vi "calc polar angles for unit vector start.vi"(10 "unit vector in":T1={"nx"=0.54, "ny"=0.6, "nz"=0.6}) -> (0 "signal valid":bool=TRUE, 1 "checksum":sgl=1.0057833, 2 "polar angles out":T2={"theta [degrees]"=53.37679, "phi [degrees]"=48.012787})   [LabVIEW 2014]
doc: "Calc Polar Angles for Unit Vector\n\nInputs a unit vector and outputs angles in polar form, while also indicating if the sensor detected a valid source.\n\nCalculations:\n\nphi = arctan(position along y-axis / position along x-axis) \ntheta = arctan (sqrt( (position along x-axis)^2 + (position along y -axis)^2) / (position along z-axis) )\nnxvalid (position along x is valid as sine or cosine) = True if -1 <= nx <= 1\nnyvalid (position along y is valid as sine or cosine) = True if -1 <= ny <= 1\nnzvalid (position along z is valid as sine or cosine) = True if -1 <= nz <= 1\n\n\n\nchecksum = sqrt( (position along x-axis)^2 + (position along y -axis)^2) / (position along z-axis)\nchecksumvalid (valid as unit 1 length) [bool] = True if 0.95 <= checksum <= 1.05, a 5% tolerance\nsignalvalid = nxvalid ^ nyvalid ^ nzvalid ^ checksumvalid\n\nBeverly Abadines\nPHY 350: E2"
uses:
  typedefs/polar angle typedef.ctl
  typedefs/unit vector typedef.ctl
panel:
  # "fully functional BD\n\nmake into a fully funtional subvi"
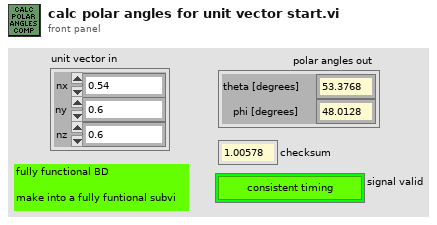
[diagram p1: front panel]
types:
  T1 = typedef "unit vector typedef.ctl" = cluster{"nx":sgl, "ny":sgl, "nz":sgl}
  T2 = typedef "polar angle typedef.ctl" = cluster{"theta [degrees]":sgl, "phi [degrees]":sgl}
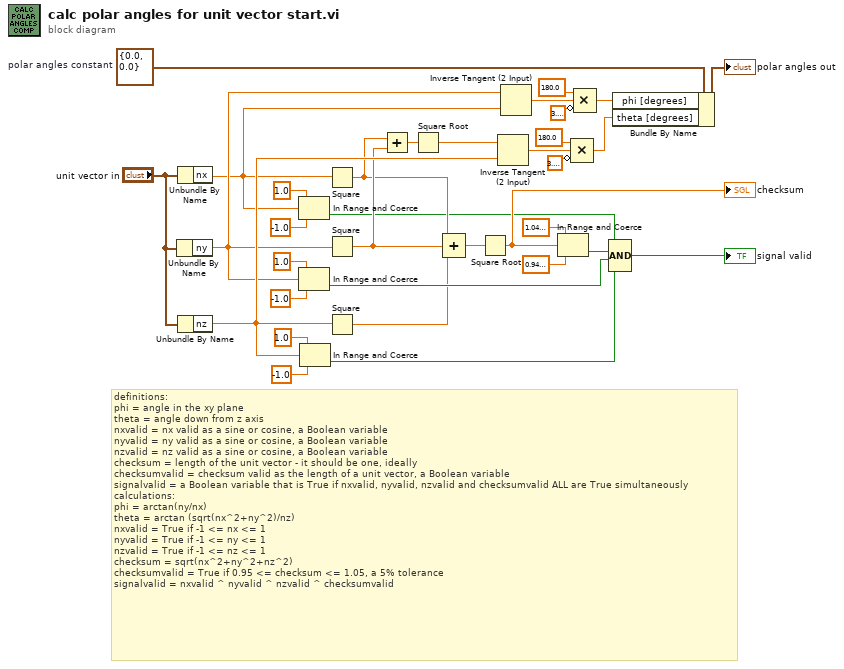
[diagram p0: block diagram]
diagram:
  w30 = T2 {"theta [degrees]"=0.0, "phi [degrees]"=0.0}  # polar angles constant
  # "definitions:\nphi = angle in the xy plane\ntheta = angle down from z axis\nnxvalid = nx valid as a sine or cosine, a Boolean variable \nnyvalid = ny valid as a sine or cosine, a Boolean variable\nnzvalid = nz valid as a sine or cosine, a Boolean variable\nchecksum = length of the unit vector - it should be one, ideally\nchecksumvalid = checksum valid as the length of a unit vector, a Boolean variable\nsignalvalid = a Boolean variable that is True if nxvalid, nyvalid, nzvalid and checksumvalid ALL are True simultaneously\ncalculations:\nphi = arctan(ny/nx)\ntheta = arctan (sqrt(nx^2+ny^2)/nz)\nnxvalid = True if -1 <= nx <= 1\nnyvalid = True if -1 <= ny <= 1\nnzvalid = True if -1 <= nz <= 1\nchecksum = sqrt(nx^2+ny^2+nz^2)\nchecksumvalid = True if 0.95 <= checksum <= 1.05, a 5% tolerance\nsignalvalid = nxvalid ^ nyvalid ^ nzvalid ^ checksumvalid"
  n1 = Unbundle By Name("unit vector in") -> ("ny"=w21:sgl)
  n2 = Unbundle By Name("unit vector in") -> ("nx"=w20:sgl)
  n3 = Unbundle By Name("unit vector in") -> ("nz"=w29:sgl)
  n4 = In Range and Coerce(upper limit=sgl 1.0, x=w20, lower limit=sgl -1.0) -> (In Range?=w15:bool)  [unwired: 1 out]
  n5 = In Range and Coerce(upper limit=sgl 1.0, x=w21, lower limit=sgl -1.0) -> (In Range?=w16:bool)  [unwired: 1 out]
  n6 = In Range and Coerce(upper limit=sgl 1.0, x=w29, lower limit=sgl -1.0) -> (In Range?=w17:bool)  [unwired: 1 out]
  n7 = Square(x=w20) -> (x^2=w22:sgl)
  n8 = Square(x=w21) -> (x^2=w23:sgl)
  n9 = Square(x=w29) -> (x^2=w11:sgl)
  n10 = Add(x=w22, y=w23) -> (x+y=w24:sgl)
  n11 = Square Root(x=w24) -> (sqrt(x)=w28:sgl)
  n12 = Compound Arithmetic op=ADD(w22, w23, w11) -> (w12:sgl)
  n13 = Square Root(x=w12) -> (sqrt(x)=w19:sgl)
  "checksum" <- w19
  n14 = Inverse Tangent (2 Input)(1:w29, 2:w28) -> (0:w27:sgl)
  n15 = Inverse Tangent (2 Input)(1:w20, 2:w21) -> (0:w1:sgl)
  n16 = In Range and Coerce(upper limit=sgl 1.05, x=w19, lower limit=sgl 0.95) -> (In Range?=w14:bool)  [unwired: 1 out]
  n17 = Compound Arithmetic op=MULTIPLY(sgl 180.0 ("value"), w27, invert sgl 3.1415927) -> (w33:sgl)
  n18 = Compound Arithmetic op=MULTIPLY(sgl 180.0 ("value"), w1, invert sgl 3.1415927) -> (w32:sgl)
  n19 = Compound Arithmetic op=AND(w15, w14, w16, w17) -> (→"signal valid":bool)
  n20 = Bundle By Name(cluster=w30, "phi [degrees]"=w32, "theta [degrees]"=w33) -> (→"polar angles out":T2)
